vi "data_array_creation(SubVI).vi"(9 "Index":dbl, 10 "Value":dbl, 11 "Array in":dbl[](array[numeric])) -> (3 "Array out":dbl[](array[numeric]))   [LabVIEW 2017]
doc: "SubVI that replace <B>Index</B> element of array with new <B>Value</B>"
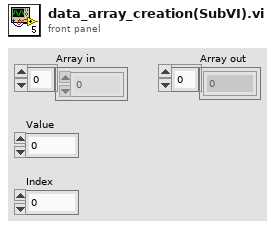
[diagram p1: front panel]
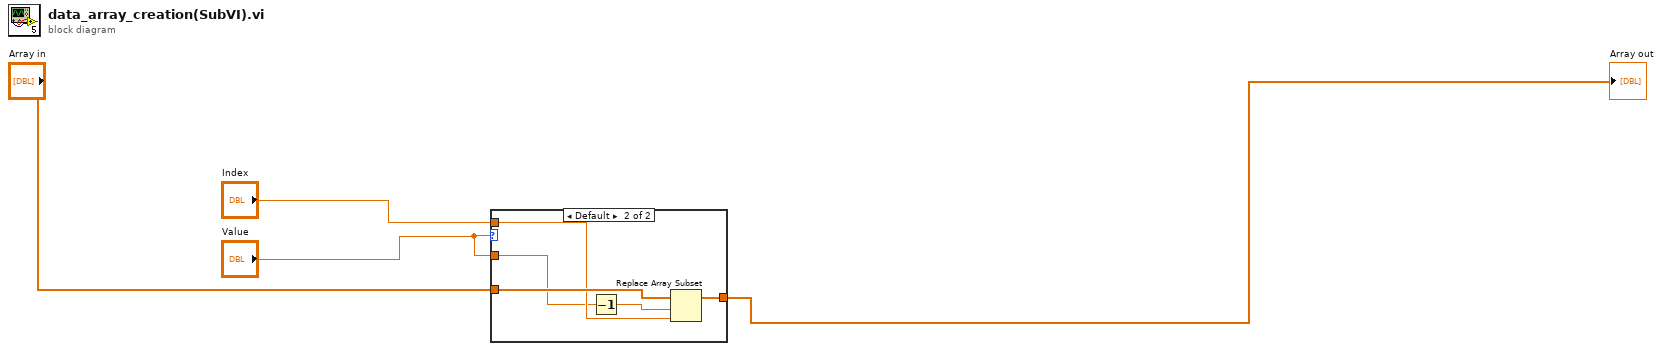
[diagram p0: block diagram]
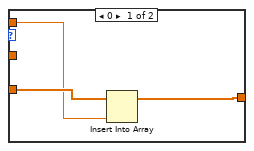
[diagram p2: hidden frame]
diagram:
  n1 = case shown="Default" "Value" {
    tunnel: "Array in" -> [w6 w12]
    tunnel: [w7 w11] -> w2
    tunnel: "Value" -> [_ w8]
    tunnel: "Index" -> [w5 w10]
    frame 0 {
      n2 = Insert Into Array(array=w6, new element=w5) -> (w7:dbl[])  [unwired: 1 in]
    }
    frame Default {
      n3 = Decrement(x=w8) -> (x-1=w9:dbl)
      n4 = Replace Array Subset(array=w12, new element=w10, index=w9) -> (w11:dbl[])
    }
  }
  "Array out" <- w2
